vi "main OP500.vi"() -> ()   [LabVIEW 2020]
uses:
  SubVI/OP500Z8_state.ctl
  ZEN8 Semi Auto EMC/OP700/SubVI/FGV/FGV_Enum.ctl
  C:/Users/elhajj/OneDrive - FORSEE POWER/Bureau/Support banc de test/Ligne ZENPLUS/Code LabVIEW/CODE/02 SLIM ZEN WS 500/SubVi/FGV.ctl
  <userlib>/PCAN Basic/Controls/BaudrateEenum.ctl
  <userlib>/PCAN Basic/Controls/Channel.ctl
  13eb9333-f902-445b-951f-98894687dcd3.vi
  4a804ed1-565a-41e0-a699-ae70de0a1211.vi
  VG/VG_progressBar.vi
  VG/VG_Barre_Progression_ISO.vi
  DiagTool/RAMPAGE V1.0/VI/CheminDeBase.vi
  VG/VG_DCIR+OUIouNON.vi
  VG/VG_OCV70min.vi
  VG/VG_OCV70max.vi
  VG/VG_OCV30max.vi
  VG/VG_OCV30min.vi
  VG/IS30%.vi
  VG/VG_ISOmin.vi
  VG/VG_DCIRmax.vi
  VG/VG_DCIRmin.vi
  <userlib>/PCAN Basic/PCANBasic.lvlib
  <userlib>/Alex_Peak_lib/PEAK_lib_ALEX.lvlib
  <vilib>/Utility/file.llb/Read Delimited Spreadsheet (string).vi
panel:
  out "Boolean":bool
  out "DCIR+ ?":bool
  out "Barre de progression ISO":dbl(slide) scale=0.0..100.0
  out "VISA OUT":T1
  out "IS30% ?":bool
  out "Cluster":T2
  out "progression":dbl(slide) scale=0.0..100.0
  out "errout":errorcluster caption="sortie d'erreur"
  out "STOP":bool
  out "TOP":string
  out "DRAW":picture
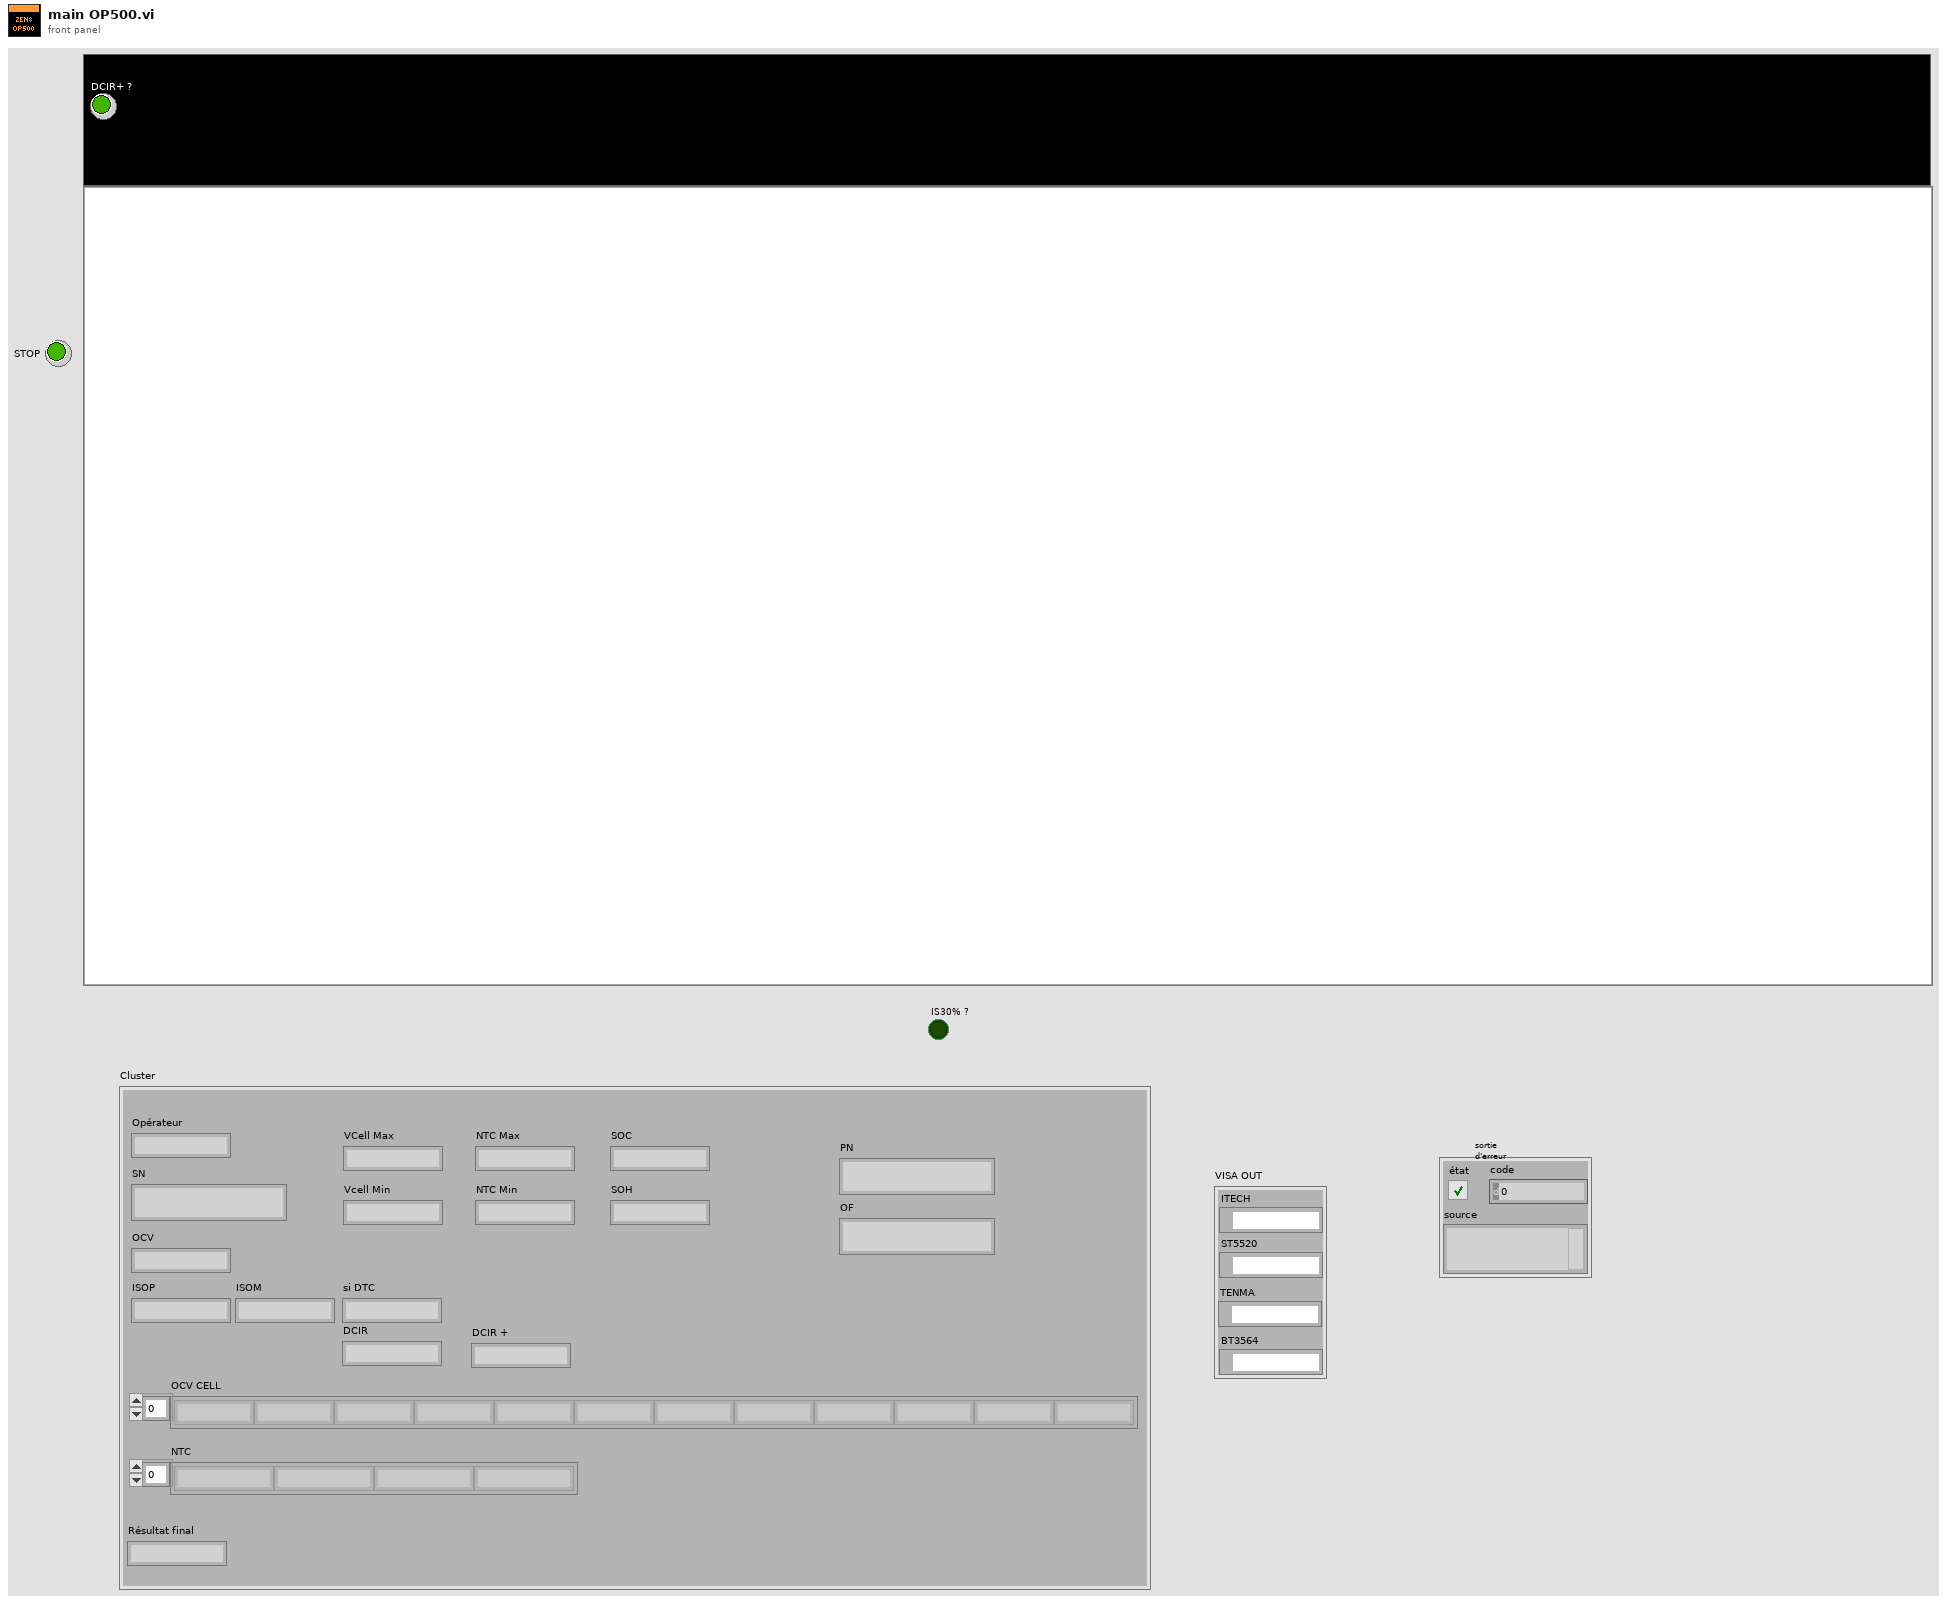
[diagram p1: front panel]
types:
  T1 = cluster{"ITECH":refnum<visa-resource-name>, "ST5520":refnum<visa-resource-name>, "TENMA":refnum<visa-resource-name>, "BT3564":refnum<visa-resource-name>}
  T2 = cluster{"Opérateur":string, "OCV":string, "ISOP":string, "ISOM":string, "Résultat final":string, "SN":string, "OCV CELL":string[], "NTC":string[], "DCIR":string, "si DTC":string, "Vcell Min":string, "VCell Max":string, "NTC Max":string, "NTC Min":string, "SOC":string, "SOH":string, "PN":string, "OF":string, "DCIR +":string}
  T3 = typedef "FGV_Enum.ctl" = enum16{"GET", "SET"}
  T4 = typedef "OP500Z8_state.ctl" = enum16{"Null", "Demarrage", "Init", "Scan", "Montage", "OCV", "Iso", "DataDyn", "Demontage", "Crash", "Next", "GoDCIR", "DCIR", "EXIT", "LogErr", "DTC"}
  T5 = typedef "FGV.ctl" = enum16{"GET", "SET", "RAZ"}
  T6 = cluster{"OCV":string, "Current":string, "VCell Max":string, "VCell Min":string, "NTC Max":string, "NTC Min":string, "SOC":string, "SOH":string, "DTC":string, "DCIR -":string, "DCIR +":string}
  T7 = cluster{"Opérateur":string, "OCV":string, "ISOP":string, "ISOM":string, "Résultat final":string, "SN":string, "OCV CELL":string[], "NTC":string[], "DCIR":string, "si DTC":string, "Vcell Min":string, "VCell Max":string, "NTC Max":string, "NTC Min":string, "SOC":string, "SOH":string, "PN":string, "OF":string, "DCIR+":string}
  T8 = typedef "imagedata.ctl" = cluster{"image type":i32, "image depth":i32, "image":u8[], "mask":u8[], "colors":u32[], "Rectangle":cluster{"left":i16, "top":i16, "right":i16, "bottom":i16}}
  T9 = typedef "PCANBasic.lvlib/Channel.ctl" = enum16{"PCAN_NONEBUS", "not used1", "not used2", "not used3", "not used4", "not used5", "not used6", "not used7", "not used8", "not used9", "not used10", "not used11", "not used12", "not used13", "not used14", "not used15", "not used16", "not used17", "not used18", "not used19", "not used20", "not used21", "not used22", "not used23", "not used24", "not used25", "not used26", "not used27", "not used28", "not used29", "not used30", "not used31", "not used32", "PCAN_ISABUS1", "PCAN_ISABUS2", "PCAN_ISABUS3", "PCAN_ISABUS4", "PCAN_ISABUS5", "PCAN_ISABUS6", "PCAN_ISABUS7", "PCAN_ISABUS8", "not used41", "not used42", "not used43", "not used44", "not used45", "not used46", "not used47", "not used48", "PCAN_DNGBUS1", "not used50", "not used51", "not used52", "not used53", "not used54", "not used55", "not used56", "not used57", "not used58", "not used59", "not used60", "not used61", "not used62", "not used63", "not used64", "PCAN_PCIBUS1", "PCAN_PCIBUS2", "PCAN_PCIBUS3", "PCAN_PCIBUS4", "PCAN_PCIBUS5", "PCAN_PCIBUS6", "PCAN_PCIBUS7", "PCAN_PCIBUS8", "not used73", "not used74", "not used75", "not used76", "not used77", "not used78", "not used79", "not used80", "PCAN_USBBUS1", "PCAN_USBBUS2", "PCAN_USBBUS3", "PCAN_USBBUS4", "PCAN_USBBUS5", "PCAN_USBBUS6", "PCAN_USBBUS7", "PCAN_USBBUS8", "Not used89", "Not used90", "Not used91", "Not used92", "Not used93", "Not used94", "Not used95", "Not used96", "PCAN_PCCBUS1", "PCAN_PCCBUS2"}
  T10 = typedef "PCANBasic.lvlib/BaudrateEenum.ctl" = enum16{"CAN_Baud_1M", "CAN_Baud_800K", "CAN_BAUD_500K", "CAN_BAUD_250K", "CAN_BAUD_125K", "CAN_BAUD_100K", "CAN_BAUD_95K", "CAN_BAUD_83K", "CAN_BAUD_50K", "CAN_BAUD_47K", "CAN_BAUD_33K", "CAN_BAUD_20K", "CAN_BAUD_10K", "CAN_BAUD_5K", "User Baudrate"}
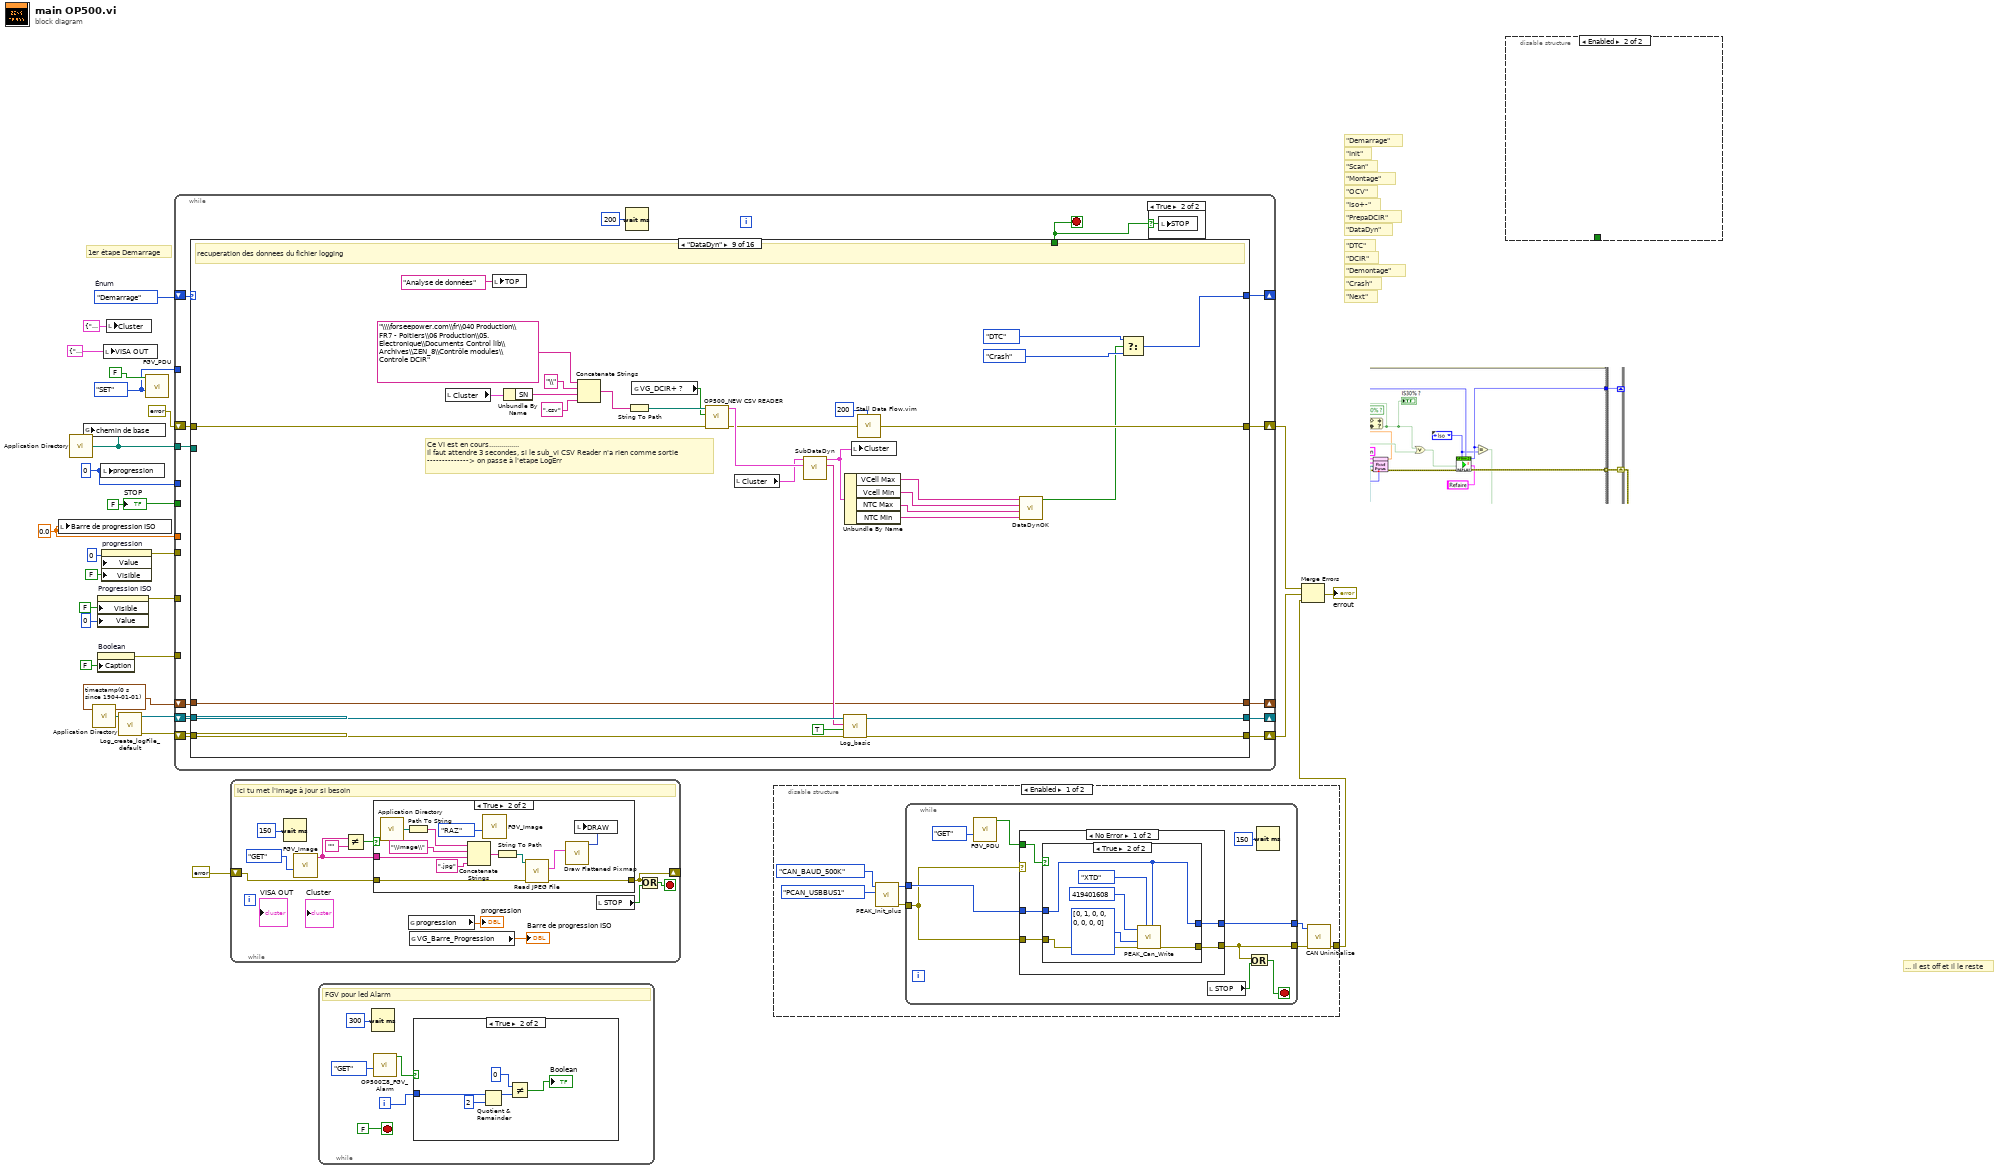
[diagram p0: block diagram]
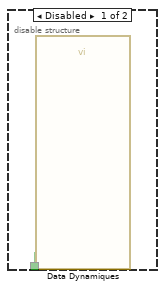
[diagram p6: hidden frame]
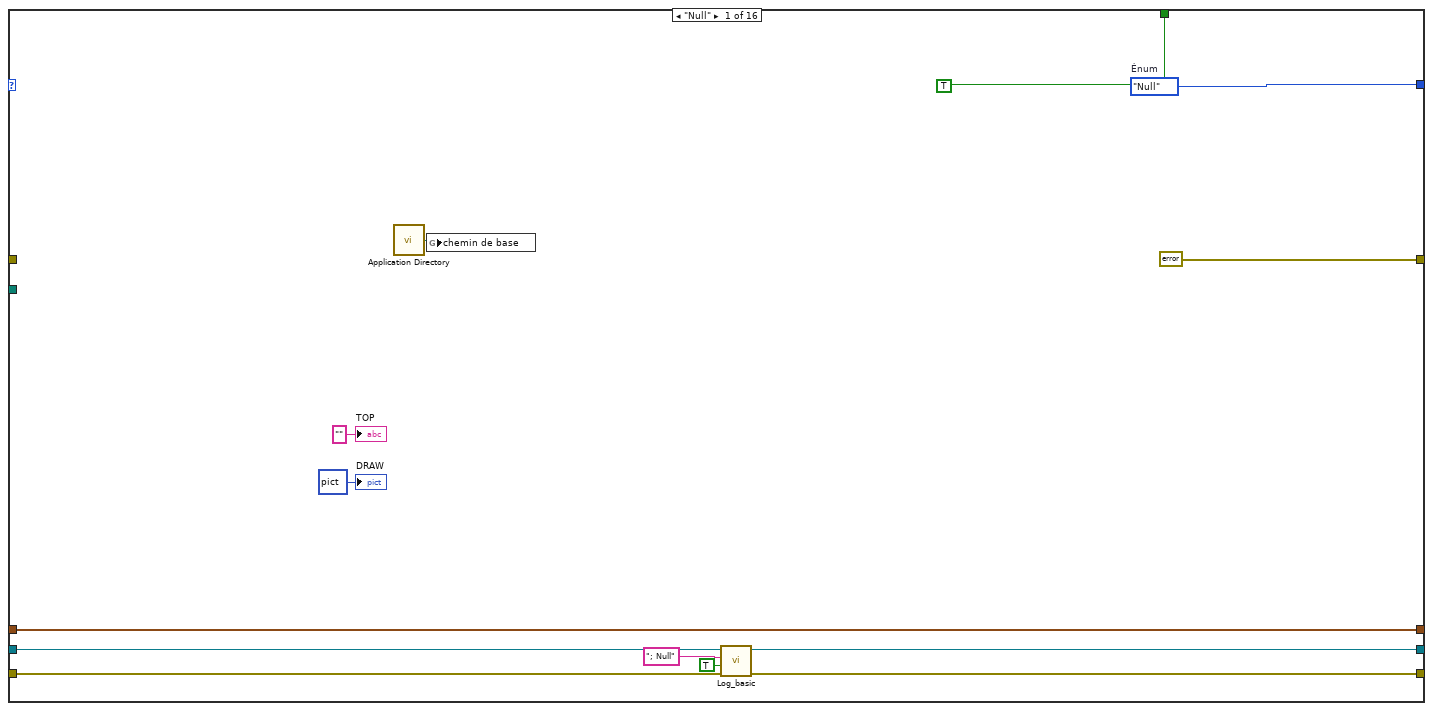
[diagram p9: hidden frame]
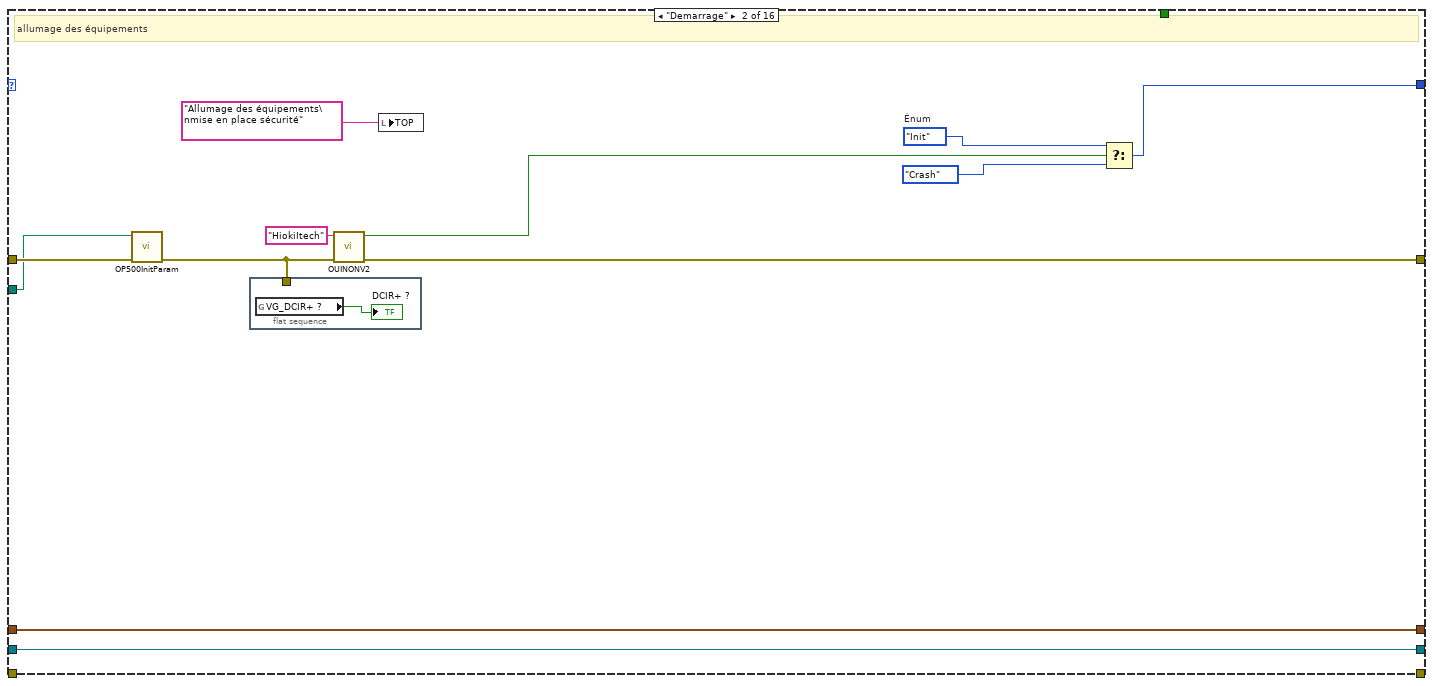
[diagram p10: hidden frame]
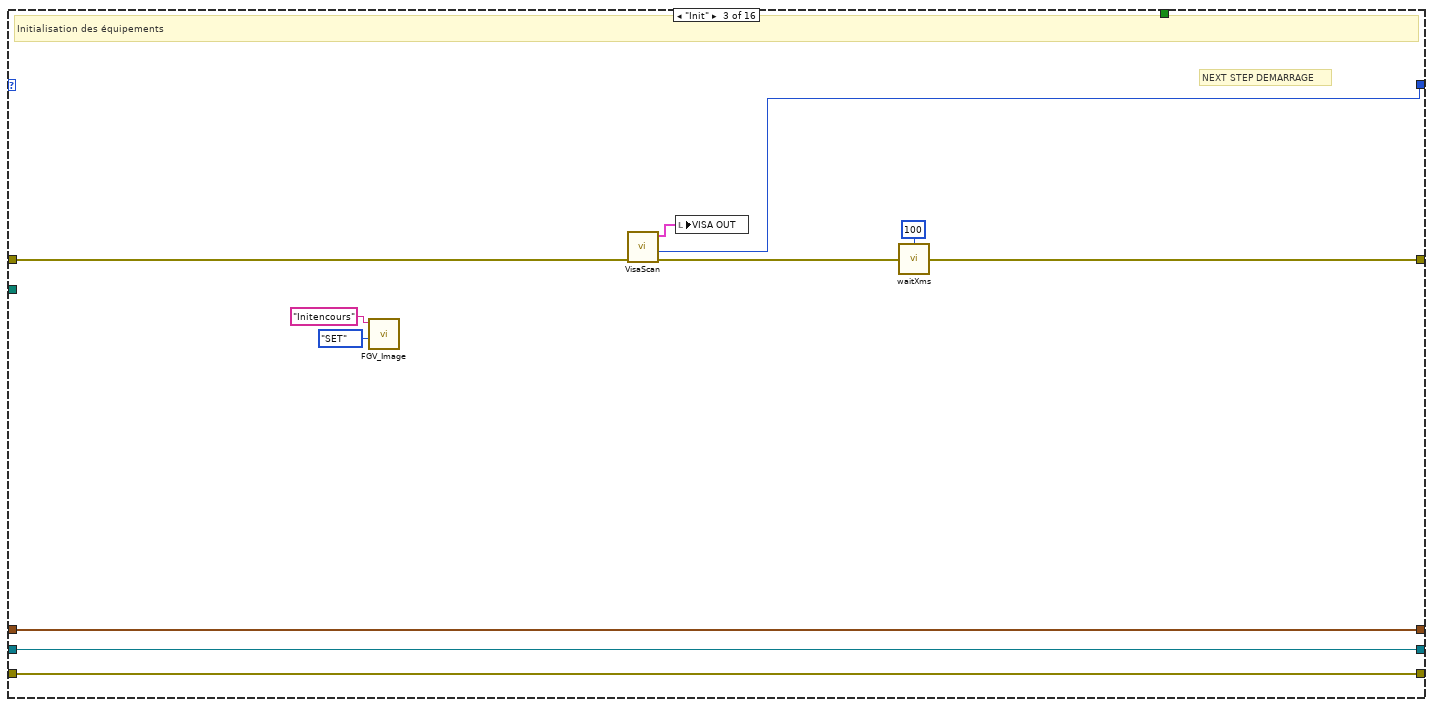
[diagram p11: hidden frame]
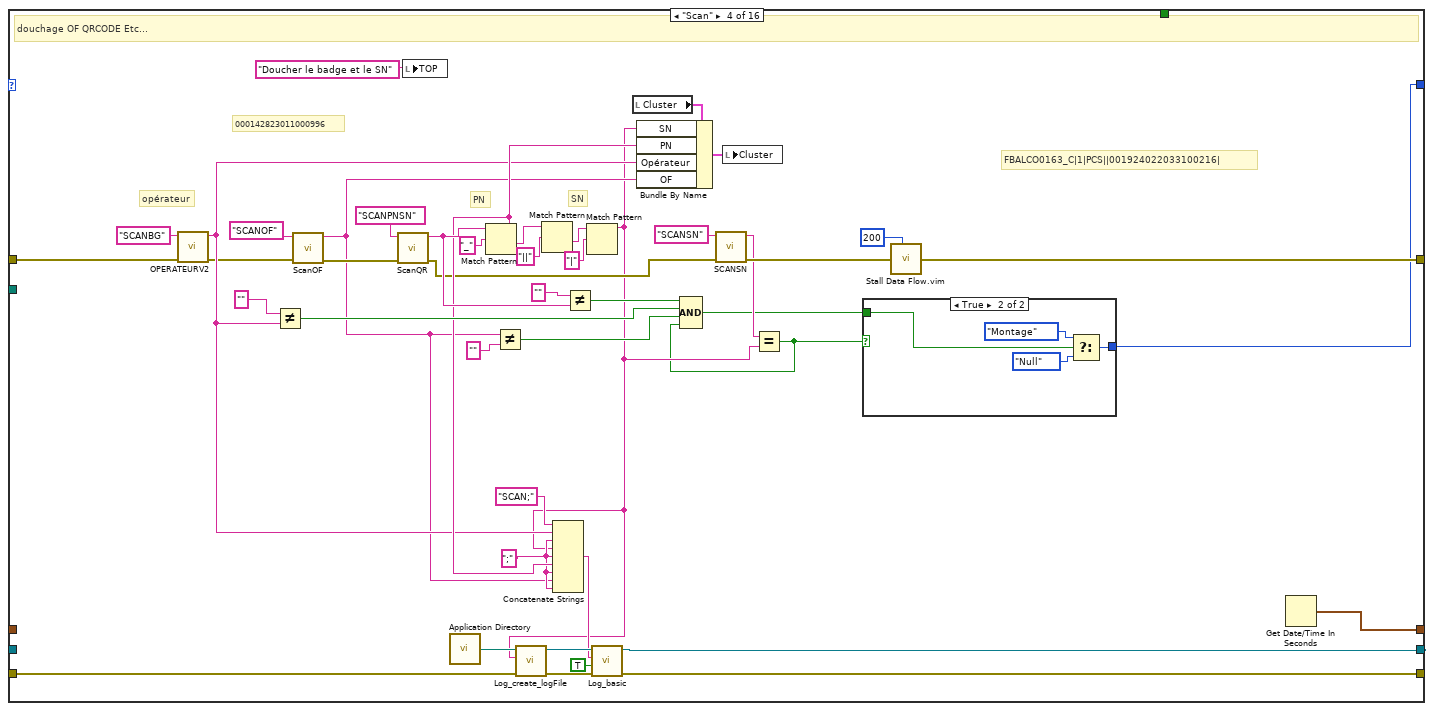
[diagram p12: hidden frame]
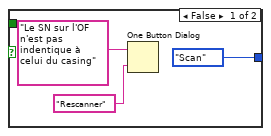
[diagram p13: hidden frame]
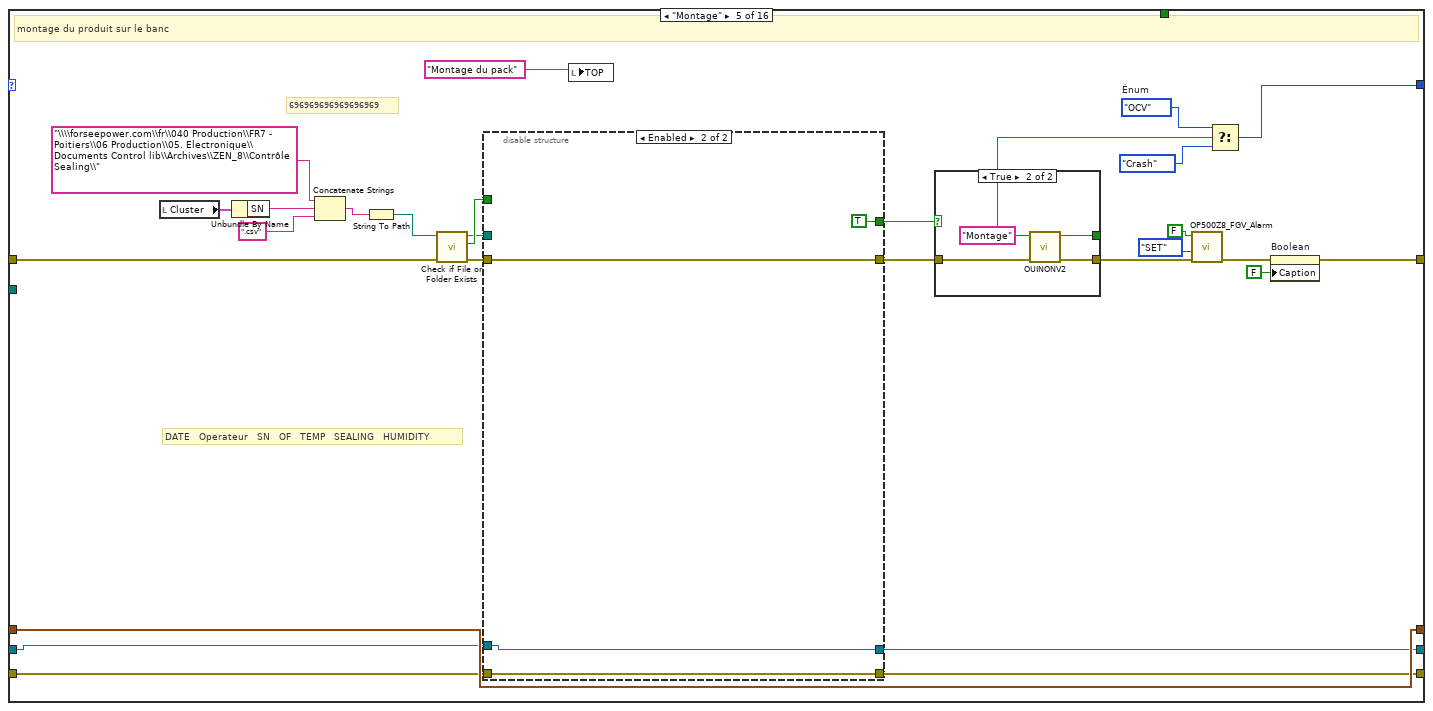
[diagram p14: hidden frame]
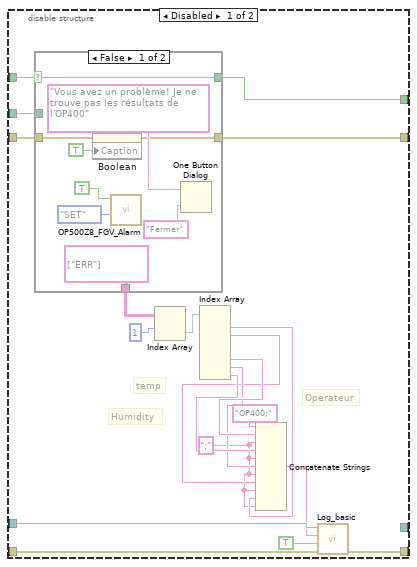
[diagram p15: hidden frame]
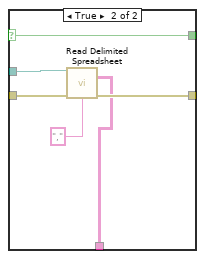
[diagram p16: hidden frame]
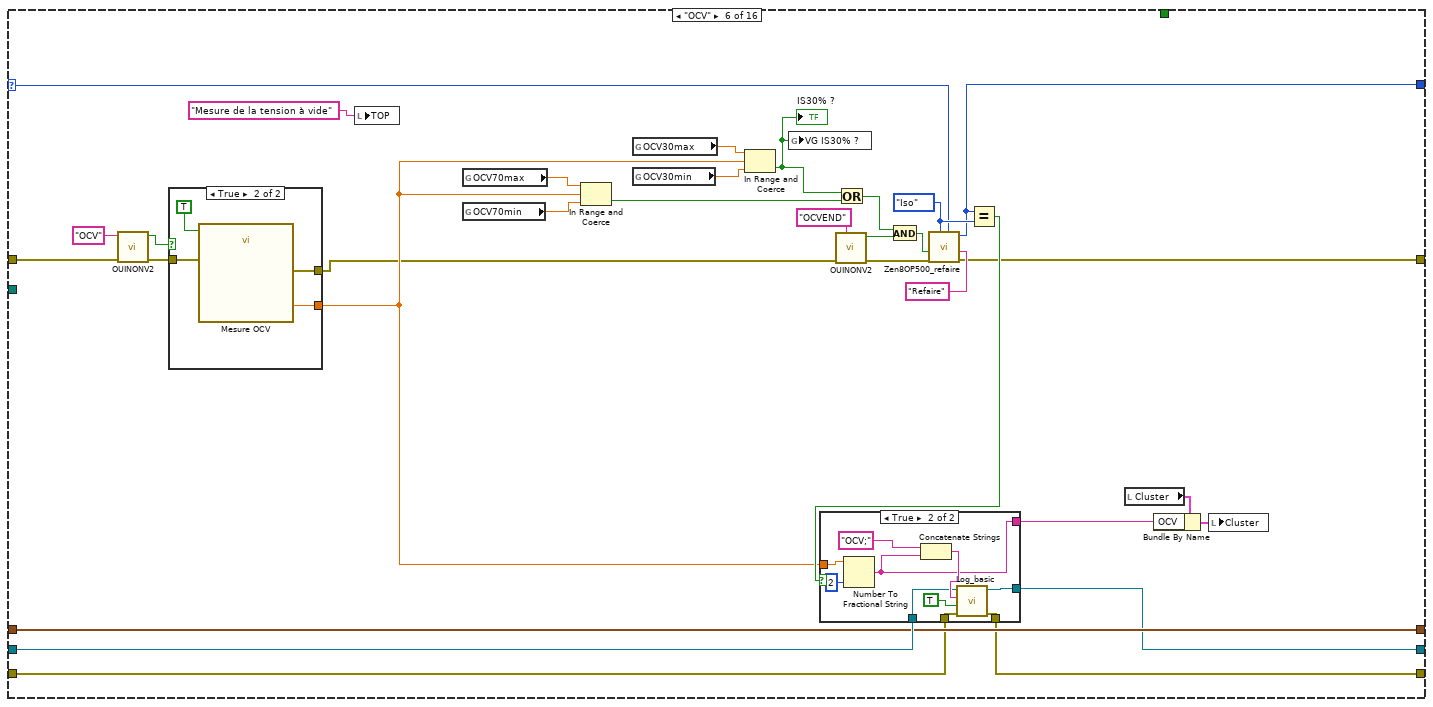
[diagram p18: hidden frame]
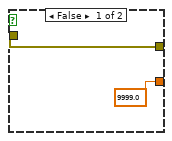
[diagram p19: hidden frame]
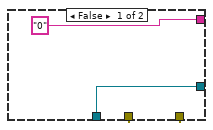
[diagram p20: hidden frame]
diagram:
  w5 = FGV_Enum."SET" ("Énum")
  w7 = 0.0 ("Barre de progression ISO")
  w17 = u8 0 ("progression")
  w12 = OP500Z8_state."Demarrage"  # Énum
  w23 = FALSE ("STOP")
  # "\"Next\""
  # "\"DCIR\""
  # "\"DTC\""
  # "1er étape Demarrage"
  # "\"Crash\""
  # "\"Demontage\""
  # "\"DataDyn\""
  # "\"Iso+-\""
  # "\"Montage\""
  # "\"Scan\""
  # "\"Init\""
  # "\"Demarrage\""
  # "\"OCV\""
  # "\"PrepaDCIR\""
  # "... il est off et il le reste"
  n1 = local write "Barre de progression ISO"(w7) -> ()
  n2 = call <vilib>:"Application Directory.vi"() -> ("Application Directory"=w22:path)
  n3 = global write "CheminDeBase.vi" "chemin de base"(w22) -> ()
  n4 = call <vilib>:"Application Directory.vi"() -> ("Application Directory"=w20:path)
  n5 = property on="Progression ISO" class="Slide (strict)"("Visible"=FALSE, "Value"=u8 0 ("Glissière")) -> (error out=w8:errorcluster)  [unwired: 2 in, 1 out]
  n6 = property on="Boolean" class="Bool (strict)"("Caption"=FALSE) -> (error out=w1:errorcluster)  [unwired: 2 in, 1 out]
  n7 = local write "progression"(w17) -> ()
  n8 = property on="progression" class="Slide (strict)"("Value"=u8 0 ("progression"), "Visible"=FALSE) -> (error out=w15:errorcluster)  [unwired: 2 in, 1 out]
  n9 = local write "VISA OUT"(T1 {"ITECH"="", "ST5520"="", "TENMA"="", "BT3564"=""} ("VISA OUT")) -> ()
  n10 = local write "Cluster"(T2 {"Opérateur"="", "OCV"="", "ISOP"="", "ISOM"="", "Résultat final"="", "SN"="", "OCV CELL"=[], "NTC"=[], "DCIR"="", "si DTC"="", "Vcell Min"="", "VCell Max"="", "NTC Max"="", "NTC Min"="", "SOC"="", "SOH"="", "PN"="", "OF"="", "DCIR +"=""} ("Cluster")) -> ()
  n11 = call <userlib>:"Log_create_logFile_default.vi"("appdir"=w20) -> ("errout"=w21:errorcluster, "Fichier à flux d'octets en sortie"=w24:refnum<file>)  [unwired: 9 in]
  n12 = call "FGV_PDU.vi"("Énum"=w5, "IN"=FALSE) -> ()  [unwired: 8 in, 2 out]
  n13 = while {
    shift-right: [w39] -> w26
    shift-left: errorcluster {"status"=FALSE, "code"=0, "source"=""} ("error out") -> [w30]
    shift-right: [w35] -> w25
    shift-left: w21 -> [w38]
    shift-right: [w36] -> _
    shift-left: w24 -> [w37]
    tunnel: w22 -> [w33]
    tunnel: w23 -> [_]
    shift-right: [w31] -> _
    shift-left: timestamp(0 s since 1904-01-01) ("seconds since 1Jan1904") -> [w32]
    tunnel: w17 -> [_]
    tunnel: w15 -> [_]
    shift-right: [w28] -> _
    shift-left: w12 -> [w29]
    tunnel: w8 -> [_]
    tunnel: w7 -> [_]
    tunnel: w5 -> [_]
    tunnel: w1 -> [_]
    stop <- w34 stop-if-true
    n14 = case "Structure Condition" shown="\"DataDyn\"" w29 {
      selector: w29 -> [_ _ _ _ _ w223 _ _ _ _ _ _ _ _ _ _]
      tunnel: w30 -> [_ w59 w73 w123 w146 w221 w272 w364 w479 w502 w528 w550 w566 w588 w640 w646]
      tunnel: [errorcluster {"status"=FALSE, "code"=0, "source"=""} ("errin") w56 w69 w89 w137 w217 w290 w359 w473 w501 w527 w544 w566 w577 w639 w647] -> w39
      tunnel: w38 -> [w50 _ w78 w119 w136 w230 w300 w365 w488 w510 w535 w552 w569 w603 _ _]
      tunnel: w37 -> [w51 w66 w77 _ w134 w232 w299 w366 w486 w509 w540 w553 w570 w604 _ _]
      tunnel: [w48 w66 w77 w121 w131 w228 w298 w366 w485 w508 w541 w553 _ _ _ _] -> w36
      tunnel: [w49 _ w78 w122 w135 w229 w301 w365 w487 w510 w542 w552 w557 w592 _ _] -> w35
      tunnel: [TRUE _ _ _ _ _ _ _ _ _ _ FALSE w571 _ _ _] -> w34
      tunnel: w33 -> [_ w58 _ _ _ _ w270 _ _ _ _ _ _ _ _ _]
      tunnel: w32 -> [w44 w65 w76 _ w158 w231 w295 w368 w478 _ _ w549 _ _ _ _]
      tunnel: [w44 w65 w76 w110 w158 w231 w295 w368 w478 _ _ w549 _ _ _ _] -> w31
      tunnel: [w42 w60 w72 w80 w153 w222 w279 w363 w465 w494 w530 w545 OP500Z8_state."Crash" w593 w636 w648] -> w28
      frame "Null" {
        w42 = OP500Z8_state."Null"  # Énum
        n15 = call <vilib>:"Application Directory.vi"() -> ("Application Directory"=w54:path)
        n16 = global write "CheminDeBase.vi" "chemin de base"(w54) -> ()
        n17 = call <userlib>:"Log_basic.vi"("errin"=w50, "date?"=TRUE, "chaîne"="; Null", "in"=w51) -> ("sortie d'erreur"=w49:errorcluster, "refnum en sortie"=w48:refnum<file>)  [unwired: 6 in]
        "DRAW" <- picture data[5B] ("DRAW")
        "TOP" <- "" ("TOP")
      }
      frame "Demarrage" {
        w62 = OP500Z8_state."Init"  # Énum
        # "allumage des équipements"
        n18 = call "OP500InitParam.vi"("errin"=w59, "pathin"=w58) -> ("errout"=w55:errorcluster)  [unwired: 9 in]
        n19 = flat-sequence {
          tunnel: w55 -> [_]
          frame #0 {
            n20 = global read "VG_DCIR+OUIouNON.vi" "VG_DCIR+ ?"() -> (→"DCIR+ ?":bool)
          }
        }
        n21 = call "OUINONV2.vi"("errin"=w55, "image"="HiokiItech") -> ("error out"=w56:errorcluster, "Booléen"=w57:bool)  [unwired: 8 in]
        n22 = local write "TOP"("Allumage des équipements\nmise en place sécurité" ("TOP")) -> ()
        n23 = Select ("Sélectionner")(t=w62, s=w57, f=OP500Z8_state."Crash" ("cas faux")) -> (s? t:f=w60:T4)
      }
      frame "Init" {
        # "NEXT STEP DEMARRAGE"
        # "Initialisation des équipements"
        n24 = call "FGV_Image.vi"("Énum"=FGV."SET", "IN"="Initencours") -> ()  [unwired: 9 in, 1 out]
        n25 = call "VisaScan.vi"("errin"=w73) -> ("errout"=w70:errorcluster, "NextStep"=w72:T4, "VISA OUT"=w68:T1)  [unwired: 8 in]
        n26 = local write "VISA OUT"(w68) -> ()
        n27 = call <userlib>:"waitXms.vi"("attente (ms)"=u32 100, "errin"=w70) -> ("errout"=w69:errorcluster)  [unwired: 13 in]
      }
      frame "Scan" {
        w93 = ";" ("chaîne")
        # "SN"
        # "PN"
        # "FBALCO0163_C|1|PCS||001924022033100216|"
        # "000142823011000996"
        # "opérateur"
        # "douchage OF QRCODE Etc..."
        n28 = call "OPERATEURV2.vi"("errin"=w123, "IN"="SCANBG") -> ("error out"=w92:errorcluster, "Dataout"=w97:string)  [unwired: 8 in]
        n29 = Not Equal?(x="", y=w97) -> (x != y?=w111:bool)
        n30 = call <userlib>:"ScanOF.vi"("errin"=w92, "image"="SCANOF") -> ("error out"=w91:errorcluster, "OF"=w87:string)  [unwired: 8 in]
        n31 = call <userlib>:"ScanQR.vi"("errin"=w91, "image"="SCANPNSN") -> ("error out"=w86:errorcluster, "OF"=w104:string)  [unwired: 7 in, 1 out]
        n32 = local write "TOP"("Doucher le badge et le SN" ("TOP")) -> ()
        n33 = call <vilib>:"Application Directory.vi"() -> ("Application Directory"=w120:path)
        n34 = Match Pattern(string=w104, regular expression="_" ("expression régulière")) -> (before substring=w98:string, after substring=w102:string)  [unwired: 1 in, 2 out]
        n35 = Not Equal?(x=w87, y="") -> (x != y?=w94:bool)
        n36 = Match Pattern(string=w102, regular expression="||" ("expression régulière")) -> (after substring=w100:string)  [unwired: 1 in, 3 out]
        n37 = Not Equal?(x="", y=w104) -> (x != y?=w112:bool)
        n38 = Match Pattern(string=w100, regular expression="|" ("expression régulière")) -> (before substring=w82:string)  [unwired: 1 in, 3 out]
        n39 = call <userlib>:"Log_create_logFile.vi"("errin"=w119, "toute l'expression"=w82, "Application Directory"=w120) -> ("sortie d'erreur"=w117:errorcluster, "Fichier à flux d'octets en sortie"=w118:refnum<file>)  [unwired: 7 in]
        n40 = Concatenate Strings("SCAN;" ("chaîne"), w97, w93, w82, w93, w98, w93, w87, w93) -> (w115:string)
        n41 = call <userlib>:"Log_basic.vi"("errin"=w117, "date?"=TRUE, "chaîne"=w115, "in"=w118) -> ("sortie d'erreur"=w122:errorcluster, "refnum en sortie"=w121:refnum<file>)  [unwired: 6 in]
        n42 = local read "Cluster"() -> (w106:T2)
        n43 = Bundle By Name(cluster=w106, "SN"=w82, "PN"=w98, "Opérateur"=w97, "OF"=w87) -> (w105:T2)
        n44 = call <userlib>:"SCANSN.vi"("errin"=w86, "image"="SCANSN") -> ("error out"=w85:errorcluster, "SN"=w83:string)  [unwired: 8 in]
        n45 = local write "Cluster"(w105) -> ()
        n46 = Equal?(x=w83, y=w82) -> (x = y?=w81:bool)
        n47 = Compound Arithmetic op=AND ("Opérateur arithmétique")(w112, w111, w94, w81) -> (w79:bool)
        n48 = case shown="True" w81 {
          tunnel: [OP500Z8_state."Scan" ("cas faux") w128] -> w80
          tunnel: w79 -> [_ w127]
          frame False {
            n49 = One Button Dialog(message="Le SN sur l'OF n'est pas indentique à celui du casing", button name ("OK")="Rescanner" ("nom du bouton (\"OK\")")) -> ()  [unwired: 1 out]
          }
          frame True {
            n50 = Select ("Sélectionner")(t=OP500Z8_state."Montage" ("Énum"), s=w127, f=OP500Z8_state."Null" ("cas faux")) -> (s? t:f=w128:T4)
          }
        }
        n51 = call "Stall Data Flow.vim"("value in"=w85, "milliseconds to wait"=u32 200) -> ("value out"=w89:errorcluster)  [unwired: 1 out]
        n52 = Get Date/Time In Seconds() -> (seconds since 1Jan1904=w110:timestamp)
      }
      frame "Montage" {
        w156 = OP500Z8_state."OCV"  # Énum
        # "DATE   Operateur   SN   OF   TEMP   SEALING   HUMIDITY"
        # "696969696969696969"
        # "montage du produit sur le banc"
        n53 = local read "Cluster"() -> (w152:T2)
        n54 = Unbundle By Name(w152) -> ("SN"=w151:string)
        n55 = Concatenate Strings("\\\\forseepower.com\\fr\\040 Production\\FR7 - Poitiers\\06 Production\\05. Electronique\\Documents Control lib\\Archives\\ZEN_8\\Contrôle Sealing\\" ("string"), w151, ".csv" ("string")) -> (w148:string)
        n56 = String To Path(string=w148) -> (path=w147:path)
        n57 = call <vilib>:"Check if File or Folder Exists.vi"("error in (no error)"=w146, "path"=w147) -> ("error out"=w145:errorcluster, "file or folder exists?"=w144:bool, "dup path"=w143:path)  [unwired: 7 in]
        n58 = disable-structure shown="Enabled" {
          disable-tunnel: w145 -> [w178 w197]
          disable-tunnel: w144 -> [w177 _]
          disable-tunnel: w143 -> [w176 _]
          disable-tunnel: w136 -> [w175 w195]
          disable-tunnel: [w174 w195] -> w135
          disable-tunnel: w134 -> [w173 w194]
          disable-tunnel: [w172 w197] -> w133
          disable-tunnel: [w171 TRUE] -> w132
          disable-tunnel: [_ w194] -> w131
          frame Disabled {
            w159 = ";" ("string")
            # "Operateur"
            # "Humidity"
            # "temp"
            n59 = case shown="False" w177 {
              selector: w177 -> [w187 w190]
              tunnel: [w182 w192] -> w172
              tunnel: w178 -> [w183 w191]
              tunnel: [w187 w190] -> w171
              tunnel: w176 -> [_ w189]
              tunnel: [string[][] [["ERR"]] ("all rows") w188] -> w166
              frame False {
                n60 = property on="Boolean" class="Bool (strict)"(error in=w183, "Caption"=TRUE) -> (error out=w182:errorcluster)  [unwired: 1 in, 1 out]
                n61 = call "OP500Z8_FGV_Alarm.vi"("Énum"=FGV_Enum."SET", "IN"=TRUE) -> ()  [unwired: 8 in, 2 out]
                n62 = One Button Dialog(message="Vous avez un problème! Je ne trouve pas les résultats de l'OP400", button name ("OK")="Fermer") -> ()  [unwired: 1 out]
              }
              frame True {
                n63 = call-poly <vilib>:"Read Delimited Spreadsheet.vi"("file path (dialog if empty)"=w189, "error in (no error)"=w191, "delimiter (\\t)"="," ("delimiter (\\t)")) -> ("all rows"=w188:string[][], "error out"=w192:errorcluster)  [unwired: 7 in, 4 out]
              }
            }
            n64 = Index Array(array=w166, index (row)=1) -> (element=w165:string[])  [unwired: 1 in]
            n65 = Index Array(array=w165) -> (element #1=w160:string, element #2=w161:string, element #5=w163:string, element #6=w162:string, element #7=w164:string)  [unwired: 7 in, 2 out]
            n66 = Concatenate Strings("OP400;" ("string"), w163, w159, w164, w159, w162, w159, w161, w159, w160, w159) -> (w169:string)
            n67 = call <userlib>:"Log_basic.vi"("errin"=w175, "date?"=TRUE, "chaîne"=w169, "in"=w173) -> ("sortie d'erreur"=w174:errorcluster)  [unwired: 6 in, 1 out]
          }
          frame Enabled {
          }
        }
        n68 = local write "TOP"("Montage du pack" ("TOP")) -> ()
        n69 = case shown="True" w132 {
          selector: w132 -> [w198 _]
          tunnel: [w199 w202] -> w142
          tunnel: [w198 w201] -> w157
          tunnel: w133 -> [w199 w200]
          frame False {
          }
          frame True {
            n70 = call "OUINONV2.vi"("errin"=w200, "image"="Montage" ("IN")) -> ("error out"=w202:errorcluster, "Booléen"=w201:bool)  [unwired: 8 in]
          }
        }
        n71 = call "OP500Z8_FGV_Alarm.vi"("errin"=w142, "Énum"=FGV_Enum."SET", "IN"=FALSE) -> ("errout"=w138:errorcluster)  [unwired: 7 in, 1 out]
        n72 = Select ("Sélectionner")(t=w156, s=w157, f=OP500Z8_state."Crash" ("cas faux")) -> (s? t:f=w153:T4)
        n73 = property on="Boolean" class="Bool (strict)"(error in=w138, "Caption"=FALSE) -> (error out=w137:errorcluster)  [unwired: 1 in, 1 out]
      }
      frame "OCV" {
        w234 = OP500Z8_state."Iso" ("Cas OK")
        n74 = call "OUINONV2.vi"("errin"=w221, "image"="OCV" ("IN")) -> ("error out"=w220:errorcluster, "Booléen"=w218:bool)  [unwired: 8 in]
        n75 = case shown="True" w218 {
          tunnel: [w237 w241] -> w213
          tunnel: [9999.0 ("Tension Bat+ Bat-") w239] -> w216
          tunnel: w220 -> [w237 w238]
          frame False {
          }
          frame True {
            n76 = call "Mesure OCV"("Enable"=TRUE, "error in (no error)"=w238) -> ("Tension Bat+ Bat-"=w239:dbl, "error out"=w241:errorcluster)  [unwired: 15 in, 1 out]
          }
        }
        n77 = local write "TOP"("Mesure de la tension à vide" ("TOP")) -> ()
        n78 = global read "VG_OCV70max.vi" "OCV70max"() -> (w207:dbl)
        n79 = global read "VG_OCV70min.vi" "OCV70min"() -> (w206:dbl)
        n80 = In Range and Coerce(upper limit=w207, x=w216, lower limit=w206) -> (In Range?=w215:bool)  [unwired: 1 out]
        n81 = global read "VG_OCV30max.vi" "OCV30max"() -> (w205:dbl)
        n82 = global read "VG_OCV30min.vi" "OCV30min"() -> (w204:dbl)
        n83 = In Range and Coerce(upper limit=w205, x=w216, lower limit=w204) -> (In Range?=w214:bool)  [unwired: 1 out]
        "IS30% ?" <- w214
        n84 = global write "IS30%.vi" "VG IS30% ?"(w214) -> ()
        n85 = call "OUINONV2.vi"("errin"=w213, "image"="OCVEND" ("IN")) -> ("error out"=w211:errorcluster, "Booléen"=w210:bool)  [unwired: 8 in]
        n86 = Or(x=w214, y=w215) -> (x .or. y?=w208:bool)
        n87 = And(x=w208, y=w210) -> (x .and. y?=w209:bool)
        n88 = call "Zen8OP500_refaire.vi"("image"="Refaire", "refaire"=w223, "casOK"=w234, "errin"=w211, "test ok ?"=w209) -> ("errout"=w217:errorcluster, "Next"=w222:T4)  [unwired: 5 in]
        n89 = Equal?(x=w222, y=w234) -> (x = y?=w233:bool)
        n90 = case shown="True" w233 {
          tunnel: w230 -> [w244 w251]
          tunnel: [w244 w250] -> w229
          tunnel: w232 -> [w243 w249]
          tunnel: [w243 w248] -> w228
          tunnel: w216 -> [_ w247]
          tunnel: ["0" w246] -> w224
          frame False {
          }
          frame True {
            n91 = Number To Fractional String(number=w247, precision (6)=i16 2 ("précision (6)")) -> (F-format string=w246:string)  [unwired: 2 in]
            n92 = Concatenate Strings("OCV;" ("chaîne"), w246) -> (w253:string)
            n93 = call <userlib>:"Log_basic.vi"("errin"=w251, "date?"=TRUE, "chaîne"=w253, "in"=w249) -> ("sortie d'erreur"=w250:errorcluster, "refnum en sortie"=w248:refnum<file>)  [unwired: 6 in]
          }
        }
        n94 = local read "Cluster"() -> (w226:T2)
        n95 = Bundle By Name(cluster=w226, "OCV"=w224) -> (w225:T2)
        n96 = local write "Cluster"(w225) -> ()
      }
      frame "Iso" {
        # "test d'isolement Bat+ et Bat-"
        n97 = call "OUINONV2.vi"("errin"=w272, "image"="ISOSTART") -> ("error out"=w277:errorcluster, "Booléen"=w275:bool)  [unwired: 8 in]
        n98 = case shown="True" w275 {
          selector: w275 -> [w308 _]
          tunnel: [w309 w313] -> w283
          tunnel: [w308 w311] -> w282
          tunnel: w277 -> [w309 w310]
          frame False {
          }
          frame True {
            n99 = call "OUINONV2.vi"("errin"=w310, "image"="MultiEPI") -> ("error out"=w313:errorcluster, "Booléen"=w311:bool)  [unwired: 8 in]
          }
        }
        n100 = local read "VISA OUT"() -> (w269:T1)
        n101 = case shown="True" w282 {
          selector: w282 -> [w314 _]
          tunnel: [w314 w318] -> w285
          tunnel: [w315 w317] -> w260
          tunnel: w283 -> [w315 w316]
          frame False {
          }
          frame True {
            n102 = call "OUINONV2.vi"("errin"=w316, "image"="ISOP" ("IN")) -> ("error out"=w317:errorcluster, "Booléen"=w318:bool)  [unwired: 8 in]
          }
        }
        n103 = Unbundle By Name(w269) -> ("ST5520"=w268:refnum<visa-resource-name>)
        n104 = global read "VG_ISOmin.vi" "Iso"() -> (w278:dbl)
        n105 = property on="PB ISO" class="Slide (strict)"(error in=w260, "Visible"=TRUE) -> (error out=w259:errorcluster)  [unwired: 1 in, 1 out]
        n106 = local write "TOP"("Test d'isolement Bat+" ("TOP")) -> ()
        n107 = case shown="True" w285 {
          selector: w285 -> [w337 _]
          tunnel: w259 -> [w338 w346]
          tunnel: [w338 w345] -> w266
          tunnel: [w336 w348] -> w297
          tunnel: [w337 w349] -> w289
          tunnel: w278 -> [_ w339]
          tunnel: [w336 w348] -> w292
          tunnel: w270 -> [_ w347]
          tunnel: w268 -> [_ w343]
          frame False {
            w336 = "ERR"
          }
          frame True {
            w350 = i16 2 ("largeur (-)")
            n108 = call "OP500Z8_ST5520.vi"("errin"=w346, "chemin de base"=w347, "Refnum VISA en entrée"=w343) -> ("error out"=w345:errorcluster, "R iso(MOhm)"=w341:dbl)  [unwired: 7 in]
            n109 = call "FGV_Image.vi"("Énum"=FGV."SET", "IN"="IsoEnCours") -> ()  [unwired: 9 in, 1 out]
            n110 = Number To Fractional String(number=w341, width (-)=w350, precision (6)=w350) -> (F-format string=w348:string)  [unwired: 1 in]
            n111 = In Range and Coerce(upper limit=9991.0 ("limite supérieure"), x=w341, lower limit=w339) -> (In Range?=w349:bool)  [unwired: 1 out]
          }
        }
        n112 = property on="PB ISO" class="Slide (strict)"(error in=w266, "Visible"=FALSE, "Value"=u8 0 ("Barre de progression ISO")) -> (error out=w264:errorcluster)  [unwired: 1 in, 1 out]
        n113 = flat-sequence {
          tunnel: w264 -> [_]
          frame #0 {
            n114 = local write "TOP"("Test d'isolement Bat-" ("TOP")) -> ()
          }
        }
        n115 = call "OUINONV2.vi"("errin"=w264, "image"="ISOM" ("IN")) -> ("error out"=w263:errorcluster, "Booléen"=w303:bool)  [unwired: 8 in]
        n116 = local read "Cluster"() -> (w294:T2)
        n117 = property on="PB ISO" class="Slide (strict)"(error in=w263, "Visible"=TRUE) -> (error out=w262:errorcluster)  [unwired: 1 in, 1 out]
        n118 = case shown="True" w303 {
          selector: w303 -> [w323 _]
          tunnel: [w321 w332] -> w257
          tunnel: [w322 w334] -> w296
          tunnel: [w323 w327] -> w288
          tunnel: w278 -> [_ w326]
          tunnel: [w322 w334] -> w291
          tunnel: w262 -> [w321 w333]
          tunnel: w270 -> [_ w331]
          tunnel: w268 -> [_ w329]
          frame False {
            w322 = "ERR"
          }
          frame True {
            w335 = i16 2 ("largeur (-)")
            n119 = call "OP500Z8_ST5520.vi"("errin"=w333, "chemin de base"=w331, "Refnum VISA en entrée"=w329) -> ("error out"=w332:errorcluster, "R iso(MOhm)"=w325:dbl)  [unwired: 7 in]
            n120 = call "FGV_Image.vi"("Énum"=FGV."SET", "IN"="IsoEnCours") -> ()  [unwired: 9 in, 1 out]
            n121 = Number To Fractional String(number=w325, width (-)=w335, precision (6)=w335) -> (F-format string=w334:string)  [unwired: 1 in]
            n122 = In Range and Coerce(upper limit=9991.0 ("limite supérieure"), x=w325, lower limit=w326) -> (In Range?=w327:bool)  [unwired: 1 out]
          }
        }
        n123 = Bundle By Name(cluster=w294, "ISOP"=w292, "ISOM"=w291) -> (w293:T2)
        n124 = local write "Cluster"(w293) -> ()
        n125 = Concatenate Strings("Iso+;" ("chaîne"), w297, ";Iso-;" ("chaîne"), w296) -> (w307:string)
        n126 = call <userlib>:"Log_basic.vi"("errin"=w300, "date?"=TRUE, "chaîne"=w307, "in"=w299) -> ("sortie d'erreur"=w301:errorcluster, "refnum en sortie"=w298:refnum<file>)  [unwired: 6 in]
        n127 = property on="PB ISO" class="Slide (strict)"(error in=w257, "Visible"=FALSE) -> (error out=w256:errorcluster)  [unwired: 1 in, 1 out]
        n128 = call "OUINONV2.vi"("errin"=w256, "image"="EPIOFF") -> ("error out"=w274:errorcluster)  [unwired: 8 in, 1 out]
        n129 = call "OUINONV2.vi"("errin"=w274, "image"="ISOEND") -> ("error out"=w290:errorcluster, "Booléen"=w287:bool)  [unwired: 8 in]
        n130 = Compound Arithmetic op=AND ("Opérateur arithmétique")(w289, w288, w287) -> (w286:bool)
        n131 = Select ("Sélectionner")(t=OP500Z8_state."GoDCIR" ("cas vrai"), s=w286, f=OP500Z8_state."Crash" ("Énum")) -> (s? t:f=w279:T4)
      }
      frame "GoDCIR" {
        # "Lancer la DCIR : fermature des contacteurs + control ITECH + Logging"
        n132 = call "OUINONV2.vi"("errin"=w364, "image"="DCIRCABLAGE") -> ("error out"=w362:errorcluster)  [unwired: 8 in, 1 out]
        n133 = local write "TOP"("Test DCIR" ("TOP")) -> ()
        n134 = local read "VISA OUT"() -> (w358:T1)
        n135 = Unbundle By Name(w358) -> ("ITECH"=w353:refnum<visa-resource-name>, "TENMA"=w352:refnum<visa-resource-name>)
        n136 = local read "Cluster"() -> (w357:T2)
        n137 = Unbundle By Name(w357) -> ("SN"=w356:string)
        n138 = disable-structure shown="Enabled" {
          disable-tunnel: w362 -> [w383 w438]
          disable-tunnel: [w380 w445] -> w361
          disable-tunnel: [w379 w446] -> w351
          disable-tunnel: w353 -> [_ w444]
          disable-tunnel: w356 -> [_ w443]
          disable-tunnel: w353 -> [_ w442]
          disable-tunnel: w352 -> [_ w437]
          frame Disabled {
            n139 = case shown="True" {
              selector: _ -> [w401 _]
              tunnel: [w401 w404] -> w374
              tunnel: w383 -> [w400 w403]
              tunnel: [w400 w402] -> w376
              frame False {
              }
              frame True {
                n140 = call "OUINONV2.vi"("errin"=w403, "image"="BMS") -> ("error out"=w402:errorcluster, "Booléen"=w404:bool)  [unwired: 8 in]
              }
            }
            n141 = case shown="True" w374 {
              selector: w374 -> [w389 _]
              tunnel: [w389 w392] -> w373
              tunnel: w376 -> [w388 w391]
              tunnel: [w388 w390] -> w375
              frame False {
              }
              frame True {
                n142 = call "OUINONV2.vi"("errin"=w391, "image"="PCANVIEW") -> ("error out"=w390:errorcluster, "Booléen"=w392:bool)  [unwired: 8 in]
              }
            }
            n143 = case shown="True" w373 {
              selector: w373 -> [w407 _]
              tunnel: [w407 w410] -> w378
              tunnel: w375 -> [w406 w409]
              tunnel: [w406 w408] -> w377
              frame False {
              }
              frame True {
                n144 = call "OUINONV2.vi"("errin"=w409, "image"="DCIRON") -> ("error out"=w408:errorcluster, "Booléen"=w410:bool)  [unwired: 8 in]
              }
            }
            n145 = case shown="True" w378 {
              selector: w378 -> [w395 _]
              tunnel: [w394 w398] -> w387
              tunnel: [w395 w397] -> w386
              tunnel: w377 -> [w394 w396]
              frame False {
              }
              frame True {
                n146 = call "OUINONV2.vi"("errin"=w396, "image"="Logging") -> ("error out"=w398:errorcluster, "Booléen"=w397:bool)  [unwired: 8 in]
              }
            }
            n147 = case shown="True" w386 {
              selector: w386 -> [w424 _]
              tunnel: w387 -> [w425 w429]
              tunnel: [w425 w427] -> w382
              tunnel: [w424 w426] -> w385
              frame False {
              }
              frame True {
                n148 = call "OUINONV2.vi"("errin"=w429, "image"="Minuteur") -> ("error out"=w427:errorcluster, "Booléen"=w426:bool)  [unwired: 8 in]
              }
            }
            n149 = case shown="True" w385 {
              selector: w385 -> [w419 _]
              tunnel: [w419 w422] -> w384
              tunnel: w382 -> [w418 w421]
              tunnel: [w418 w420] -> w381
              frame False {
              }
              frame True {
                n150 = call "OUINONV2.vi"("errin"=w421, "image"="Decharge") -> ("error out"=w420:errorcluster, "Booléen"=w422:bool)  [unwired: 8 in]
              }
            }
            n151 = case shown="True" w384 {
              selector: w384 -> [w413 _]
              tunnel: [w413 w416] -> w380
              tunnel: w381 -> [w412 w415]
              tunnel: [w412 w414] -> w379
              frame False {
              }
              frame True {
                n152 = call "OUINONV2.vi"("errin"=w415, "image"="StopLogging") -> ("error out"=w414:errorcluster, "Booléen"=w416:bool)  [unwired: 8 in]
              }
            }
          }
          frame Enabled {
            n153 = call "TENMA_Conf_On.vi"("errin"=w438, "Visa in tenma"=w437) -> ("sortie d'erreur"=w432:errorcluster)  [unwired: 9 in]
            n154 = call "FGV_PDU.vi"("errin"=w432, "Énum"=FGV_Enum."SET", "IN"=TRUE) -> ("errout"=w431:errorcluster)  [unwired: 7 in, 1 out]
            n155 = call <userlib>:"waitXms.vi"("attente (ms)"=u32 600, "errin"=w431) -> ("errout"=w436:errorcluster)  [unwired: 13 in]
            n156 = call "VerifPreDCIR.vi"("errin"=w436, "VISA resource name"=w442) -> ("errout"=w440:errorcluster, "V>35 ?"=w430:bool)  [unwired: 8 in]
            n157 = call <userlib>:"waitXms.vi"("attente (ms)"=u32 600, "errin"=w440) -> ("errout"=w439:errorcluster)  [unwired: 13 in]
            n158 = case shown="True" w430 {
              selector: w430 -> [w449 _]
              tunnel: [w448 w451] -> w446
              tunnel: [w449 w456] -> w445
              tunnel: w444 -> [_ w455]
              tunnel: w443 -> [_ w454]
              tunnel: w439 -> [w448 w458]
              frame False {
                n159 = One Button Dialog(message="Vérifier le branchement de la com, \net que le bouton du tiroir est bien sur DCIR ") -> ()  [unwired: 1 in, 1 out]
              }
              frame True {
                n160 = property on="progression" class="Slide (strict)"(error in=w458, "Visible"=TRUE) -> (error out=w457:errorcluster)  [unwired: 1 in, 1 out]
                n161 = flat-sequence {
                  tunnel: w457 -> [_]
                  frame #0 {
                    n162 = call "FGV_Image.vi"("Énum"=FGV."SET", "IN"="DCIR-EnCours") -> ()  [unwired: 9 in, 1 out]
                  }
                }
                n163 = call "OP500Z8M_ReadFromPDU.vi"("errin"=w457, "SN"=w454, "VISA ITECH Name ?"=w455) -> ("errout"=w450:errorcluster, "BMS OK ?"=w456:bool)  [unwired: 6 in, 1 out]
                n164 = call "FGV_PDU.vi"("errin"=w450, "Énum"=FGV_Enum."SET", "IN"=FALSE) -> ("errout"=w451:errorcluster)  [unwired: 7 in, 1 out]
              }
            }
          }
        }
        n165 = flat-sequence {
          tunnel: [w372] -> w363
          tunnel: w361 -> [w369]
          tunnel: w359 -> [_]
          frame #0 {
            n166 = Select(t=OP500Z8_state."DataDyn" ("Énum"), s=w369, f=OP500Z8_state."GoDCIR" ("cas faux")) -> (s? t:f=w372:T4)
          }
        }
        n167 = property on="progression" class="Slide (strict)"(error in=w351, "Visible"=FALSE, "Value"=0.0 ("progression")) -> (error out=w359:errorcluster)  [unwired: 1 in, 1 out]
      }
      frame "DataDyn" {
        # "Ce VI est en cours...............\nIl faut attendre 3 secondes, si le sub_vi CSV Reader n'a rien comme sortie\n--------------> on passe à l'etape LogErr"
        # "recuperation des donnees du fichier logging"
        n168 = local read "Cluster"() -> (w492:T2)
        n169 = local write "TOP"("Analyse de données" ("TOP")) -> ()
        n170 = Unbundle By Name(w492) -> ("SN"=w489:string)
        n171 = Concatenate Strings("\\\\forseepower.com\\fr\\040 Production\\FR7 - Poitiers\\06 Production\\05. Electronique\\Documents Control lib\\Archives\\ZEN_8\\Contrôle modules\\Controle DCIR", "\\" ("chaîne"), w489, ".csv" ("chaîne")) -> (w476:string)
        n172 = String To Path(string=w476) -> (path=w480:path)
        n173 = global read "VG_DCIR+OUIouNON.vi" "VG_DCIR+ ?"() -> (w462:bool)
        n174 = call "OP500_NEW CSV READER.vi"("errin"=w479, "DCIR+ ?"=w462, "Choisir le fichier CSV"=w480) -> ("sortie d'erreur"=w474:errorcluster, "cluster"=w477:T6)  [unwired: 5 in]
        n175 = local read "Cluster"() -> (w472:T2)
        n176 = call "SubDataDyn.vi"("cluster"=w477, "Cluster en entrée"=w472) -> ("Chaîne"=w482:string, "cluster de sortie"=w471:T7)  [unwired: 8 in]
        n177 = call <userlib>:"Log_basic.vi"("errin"=w488, "date?"=TRUE, "chaîne"=w482, "in"=w486) -> ("sortie d'erreur"=w487:errorcluster, "refnum en sortie"=w485:refnum<file>)  [unwired: 6 in]
        n178 = Unbundle By Name(w471) -> ("VCell Max"=w470:string, "Vcell Min"=w469:string, "NTC Max"=w467:string, "NTC Min"=w468:string)
        n179 = local write "Cluster"(w471) -> ()
        n180 = call "Stall Data Flow.vim"("value in"=w474, "milliseconds to wait"=u32 200) -> ("value out"=w473:errorcluster)  [unwired: 1 out]
        n181 = call "DataDynOK"("NTC Min"=w468, "NTC Max"=w467, "Vcell Min"=w469, "VCell Max"=w470) -> ("DataDynOK ?"=w463:bool)  [unwired: 7 in]
        n182 = Select(t=OP500Z8_state."DTC" ("Next"), s=w463, f=OP500Z8_state."Crash" ("cas faux")) -> (s? t:f=w465:T4)
      }
      frame "DTC" {
        w499 = ";" ("chaîne")
        # "Voir s'il Y a des DTC"
        n183 = local write "TOP"("Analyse les DTC" ("TOP")) -> ()
        n184 = local read "Cluster"() -> (w504:T2)
        n185 = Unbundle By Name(w504) -> ("si DTC"=w498:string)
        n186 = Equal?(x="NO DTC", y=w498) -> (x = y?=w496:bool)
        n187 = call <userlib>:"waitXms.vi"("attente (ms)"=u32 100, "errin"=w502) -> ("errout"=w501:errorcluster)  [unwired: 13 in]
        n188 = Concatenate Strings("DTC" ("chaîne"), w499, w498, w499) -> (w505:string)
        n189 = call <userlib>:"Log_basic.vi"("date?"=TRUE, "chaîne"=w505, "in"=w509) -> ("refnum en sortie"=w508:refnum<file>)  [unwired: 7 in, 1 out]
        n190 = Select(t=OP500Z8_state."DCIR" ("Énum"), s=w496, f=OP500Z8_state."Crash" ("cas faux")) -> (s? t:f=w494:T4)
      }
      frame "DCIR" {
        w519 = ";" ("chaîne")
        # "Recuperation de la valeur DCIR"
        n191 = local write "TOP"("Calcule de la resistance interne" ("TOP")) -> ()
        n192 = local read "Cluster"() -> (w536:T2)
        n193 = global read "VG_DCIR+OUIouNON.vi" "VG_DCIR+ ?"() -> (w516:bool)
        n194 = Unbundle By Name(w536) -> ("DCIR"=w534:string, "DCIR +"=w515:string)
        n195 = call <userlib>:"waitXms.vi"("attente (ms)"=u32 100, "errin"=w528) -> ("errout"=w527:errorcluster)  [unwired: 13 in]
        n196 = Select(t=w515, s=w516, f="NA") -> (s? t:f=w517:string)
        n197 = Concatenate Strings("DCIR-" ("chaîne"), w519, w534, w519, "DCIR+" ("string"), w519, w517, w519) -> (w538:string)
        n198 = Fract/Exp String To Number(string=w534) -> (number=w533:dbl)  [unwired: 3 in, 1 out]
        n199 = call <userlib>:"Log_basic.vi"("errin"=w535, "date?"=TRUE, "chaîne"=w538, "in"=w540) -> ("sortie d'erreur"=w542:errorcluster, "refnum en sortie"=w541:refnum<file>)  [unwired: 6 in]
        n200 = global read "VG_DCIRmax.vi" "DCIRmax"() -> (w524:dbl)
        n201 = global read "VG_DCIRmin.vi" "DCIRmin"() -> (w513:dbl)
        n202 = Increment(x=w513) -> (x+1=w512:dbl)
        n203 = Number To Decimal String(number=w512) -> (decimal integer string=w511:string)  [unwired: 1 in]
        n204 = Select(t=w515, s=w516, f=w511) -> (s? t:f=w514:string)
        n205 = Fract/Exp String To Number(string=w514) -> (number=w525:dbl)  [unwired: 3 in, 1 out]
        n206 = In Range and Coerce(upper limit=w524, x=w533, lower limit=w513) -> (In Range?=w523:bool)  [unwired: 1 out]
        n207 = In Range and Coerce(upper limit=w524, x=w525, lower limit=w513) -> (In Range?=w522:bool)  [unwired: 1 out]
        n208 = And(x=w523, y=w522) -> (x .and. y?=w521:bool)
        n209 = Select(t=OP500Z8_state."Demontage" ("Énum"), s=w521, f=OP500Z8_state."Crash" ("Énum")) -> (s? t:f=w530:T4)
      }
      frame "Demontage" {
        w548 = OP500Z8_state."Next"  # Énum
        n210 = local write "TOP"("Demontage du pack" ("TOP")) -> ()
        n211 = call "OUINONV2.vi"("errin"=w550, "image"="Demontage2" ("IN")) -> ("error out"=w544:errorcluster, "Booléen"=w543:bool)  [unwired: 8 in]
        n212 = Select ("Sélectionner")(t=w548, s=w543, f=OP500Z8_state."Demontage" ("cas faux")) -> (s? t:f=w545:T4)
      }
      frame "Crash" {
        w556 = path "\\\\forseepower.com\\fr/040 Production/FR7 - Poitiers/06 Production/05. Electronique/Documents Control lib/Archives/ZEN_8/Contrôle modules/PV OP500" ("chemin de la cible (utiliser une boîte de dialogue)")
        # "C:\\Users\\ELHAJJ\\OneDrive - FORSEE POWER\\Bureau\\PV ZEN8 TEST"
        n213 = Close File(refnum=w570, error in=w569) -> (path=w559:path, error out=w562:errorcluster)
        n214 = call <userlib>:"waitXms.vi"("attente (ms)"=u32 300, "errin"=w562) -> ("errout"=w560:errorcluster)  [unwired: 13 in]
        n215 = Read from Text File(file (use dialog)=w559, error in=w560) -> (error out=w555:errorcluster)  [unwired: 2 in, 3 out]
        n216 = call "FGV_Image.vi"("Énum"=FGV."SET", "IN"="Crash") -> ()  [unwired: 9 in, 1 out]
        n217 = Copy ("Copier")(8:w555, 10:w556, 11:w559) -> (0:w561:errorcluster)  [unwired: 2 in, 2 out]
        n218 = call "PvgeneratorOP500.vi"("errin"=w561, "network"=w556, "path in"=w559) -> ("sortie d'erreur"=w565:errorcluster, "network out"=w564:path)  [unwired: 5 in, 2 out]
        n219 = call <userlib>:"POP_GOOGLE.vi"("error in"=w565, "chemin"=w564) -> ("error out"=w557:errorcluster)  [unwired: 8 in, 1 out]
        n220 = flat-sequence {
          tunnel: [TRUE] -> w571
          tunnel: w557 -> [_]
          frame #0 {
          }
        }
      }
      frame "Next" {
        w591 = path "\\\\forseepower.com\\fr/040 Production/FR7 - Poitiers/06 Production/05. Electronique/Documents Control lib/Archives/ZEN_8/Contrôle modules/PV OP500" ("chemin de la cible (utiliser une boîte de dialogue)")
        w601 = OP500Z8_state."EXIT"  # Énum
        w602 = OP500Z8_state."Scan"  # Énum
        n221 = global read "VG_DCIR+OUIouNON.vi" "VG_DCIR+ ?"() -> (w576:bool)
        n222 = Select(t="PassNbMP" ("IN"), s=w576, f="PassNbM") -> (s? t:f=w573:string)
        n223 = call "OUINONV2.vi"("errin"=w588, "image"=w573) -> ("error out"=w587:errorcluster, "Booléen"=w586:bool)  [unwired: 8 in]
        n224 = Close File(refnum=w604, error in=w603) -> (path=w594:path, error out=w600:errorcluster)
        n225 = case shown="True" w586 {
          selector: w586 -> [w623 _]
          tunnel: w587 -> [w624 w627]
          tunnel: [w623 w626] -> w584
          tunnel: [w624 w625] -> w583
          frame False {
          }
          frame True {
            n226 = call "OUINONV2.vi"("errin"=w627, "image"="EttJaune" ("IN")) -> ("error out"=w625:errorcluster, "Booléen"=w626:bool)  [unwired: 8 in]
          }
        }
        n227 = call <userlib>:"waitXms.vi"("attente (ms)"=u32 300, "errin"=w600) -> ("errout"=w596:errorcluster)  [unwired: 13 in]
        n228 = Read from Text File(file (use dialog)=w594, error in=w596) -> (error out=w590:errorcluster)  [unwired: 2 in, 3 out]
        n229 = case shown="True" w584 {
          selector: w584 -> [w618 _]
          tunnel: w583 -> [w617 w621]
          tunnel: [w618 w620] -> w585
          tunnel: [w617 w619] -> w582
          frame False {
          }
          frame True {
            n230 = call "OUINONV2.vi"("errin"=w621, "image"="EttBleu" ("IN")) -> ("error out"=w619:errorcluster, "Booléen"=w620:bool)  [unwired: 8 in]
          }
        }
        n231 = case shown="True" w585 {
          selector: w585 -> [w612 _]
          tunnel: w582 -> [w611 w615]
          tunnel: [w612 w614] -> w579
          tunnel: [w611 w613] -> w581
          frame False {
          }
          frame True {
            n232 = call "OUINONV2.vi"("errin"=w615, "image"="eProd" ("IN")) -> ("error out"=w613:errorcluster, "Booléen"=w614:bool)  [unwired: 8 in]
          }
        }
        n233 = Copy ("Copier")(8:w590, 10:w591, 11:w594) -> (0:w595:errorcluster)  [unwired: 2 in, 2 out]
        n234 = call "PvgeneratorOP500.vi"("errin"=w595, "network"=w591, "path in"=w594) -> ("sortie d'erreur"=w598:errorcluster, "network out"=w597:path)  [unwired: 5 in, 2 out]
        n235 = case shown="True" w579 {
          selector: w579 -> [w606 _]
          tunnel: w581 -> [w605 w609]
          tunnel: [w606 w608] -> w578
          tunnel: [w605 w607] -> w580
          frame False {
          }
          frame True {
            n236 = call "OUINONV2.vi"("errin"=w609, "image"="ProdOF" ("IN")) -> ("error out"=w607:errorcluster, "Booléen"=w608:bool)  [unwired: 8 in]
          }
        }
        n237 = call <userlib>:"POP_GOOGLE.vi"("error in"=w598, "chemin"=w597) -> ("error out"=w592:errorcluster)  [unwired: 8 in, 1 out]
        n238 = case shown="True" w578 {
          selector: w578 -> [w630 _]
          tunnel: [w629 w633] -> w577
          tunnel: w580 -> [w629 w631]
          tunnel: [w630 w632] -> w589
          frame False {
          }
          frame True {
            n239 = call "OUINONV2.vi"("errin"=w631, "image"="Next" ("IN")) -> ("error out"=w633:errorcluster, "Booléen"=w632:bool)  [unwired: 8 in]
          }
        }
        n240 = Select(t=w602, s=w589, f=w601) -> (s? t:f=w593:T4)
      }
      frame "EXIT" {
        # "Eteindre le banc avant de quitter labview"
        n241 = call "OUINONV2.vi"("errin"=w640, "image"="TurnOff" ("IN")) -> ("error out"=w639:errorcluster, "Booléen"=w638:bool)  [unwired: 8 in]
        n242 = Select(t=OP500Z8_state."EXIT" ("cas vrai"), s=w638, f=OP500Z8_state."Null" ("Énum")) -> (s? t:f=w636:T4)
        n243 = flat-sequence {
          tunnel: w639 -> [_]
          frame #0 {
            n244 = Quit LabVIEW(quit? (T)=TRUE ("quitter ? (V)")) -> ()
          }
        }
      }
      frame "LogErr" {
        # "En cours.................................................................................................."
        # "au cas ou le fichier de log n'existe pas ou il contient pas le test DCIR"
        n245 = call "OUINONV2.vi"("errin"=w646, "image"="LogErr") -> ("error out"=w647:errorcluster, "Booléen"=w645:bool)  [unwired: 8 in]
        n246 = Select(t=OP500Z8_state."GoDCIR" ("cas vrai"), s=w645, f=OP500Z8_state."Crash" ("Énum")) -> (s? t:f=w648:T4)
      }
    }
    n247 = Wait (ms)(milliseconds to wait=u32 200 ("attente (ms)")) -> ()  [unwired: 1 out]
    n248 = case shown="True" w34 {
      selector: w34 -> [_ w41]
      frame False {
      }
      frame True {
        n249 = local write "STOP"(w41) -> ()
      }
    }
  }
  n250 = while {
    shift-right: [w659] -> _
    shift-left: errorcluster {"status"=FALSE, "code"=0, "source"=""} ("error out") -> [w656]
    stop <- w657 stop-if-true
    # "ici tu met l'image à jour si besoin"
    n251 = Wait (ms)(milliseconds to wait=u32 150 ("attente (ms)")) -> ()  [unwired: 1 out]
    n252 = call "FGV_Image.vi"("Énum"=FGV."GET") -> ("OUT"=w652:string)  [unwired: 10 in]
    n253 = Not Equal?(x=w652, y="") -> (x != y?=w653:bool)
    n254 = case shown="True" w653 {
      tunnel: [w661 w666] -> w659
      tunnel: w656 -> [w661 w665]
      tunnel: w652 -> [_ w664]
      frame False {
      }
      frame True {
        n255 = call <vilib>:"Application Directory.vi"() -> ("Application Directory"=w669:path)
        n256 = Path To String(path=w669) -> (string=w670:string)
        n257 = Concatenate Strings(w670, "\\Image\\" ("chaîne"), w664, ".jpg" ("chaîne")) -> (w668:string)
        n258 = call "FGV_Image.vi"("Énum"=FGV."RAZ") -> ()  [unwired: 10 in, 1 out]
        n259 = String To Path(string=w668) -> (path=w667:path)
        n260 = call <vilib>:"Read JPEG File.vi"("error in (no error)"=w665, "path to JPEG file"=w667) -> ("error out"=w666:errorcluster, "image data"=w673:T8)  [unwired: 7 in, 1 out]
        n261 = call <vilib>:"Draw Flattened Pixmap.vi"("image data"=w673) -> ("new picture"=w662:picture)  [unwired: 8 in]
        n262 = local write "DRAW"(w662) -> ()
      }
    }
    n263 = global read "VG_progressBar.vi" "progression"() -> (→"progression":dbl)
    n264 = global read "VG_Barre_Progression_ISO.vi" "VG_Barre_Progression"() -> (→"Barre de progression ISO":dbl)
    n265 = local read "STOP"() -> (w658:bool)
    n266 = Or(x=w659, y=w658) -> (x .or. y?=w657:bool)
  }
  n267 = while {
    i -> [w676]
    stop <- FALSE stop-if-true
    # "FGV pour led Alarm"
    n268 = Wait (ms)(milliseconds to wait=u32 300) -> ()  [unwired: 1 out]
    n269 = call "OP500Z8_FGV_Alarm.vi"("Énum"=FGV_Enum."GET") -> ("OUT"=w674:bool)  [unwired: 9 in, 1 out]
    n270 = case shown="True" w674 {
      tunnel: w676 -> [_ w679]
      frame False {
      }
      frame True {
        n271 = Quotient & Remainder(x=w679, y=2) -> (x-y*floor(x/y)=w682:i32)  [unwired: 1 out]
        n272 = Not Equal?(x=0, y=w682) -> (x != y?=→"Boolean":bool)
      }
    }
  }
  n273 = disable-structure shown="Enabled" {
    disable-tunnel: [w684 _] -> w4
    frame Enabled {
      n274 = call <userlib>:"PEAK_Init_plus.vi"("Channel"=Channel."PCAN_USBBUS1", "BTR0BTR1"=BaudrateEenum."CAN_BAUD_500K") -> ("errout"=w688:errorcluster, "Channel out"=w687:T9)  [unwired: 8 in]
      n275 = while {
        tunnel: w688 -> [w692]
        tunnel: w687 -> [w697]
        tunnel: [w694] -> w686
        tunnel: [w696] -> w685
        stop <- w695 stop-if-true
        n276 = call "FGV_PDU.vi"("Énum"=FGV_Enum."GET") -> ("OUT"=w698:bool)  [unwired: 9 in, 1 out]
        n277 = case shown="No Error" w692 {
          tunnel: w698 -> [w704 _]
          tunnel: w692 -> [w703 w714]
          tunnel: w697 -> [w702 w713]
          tunnel: [w701 w713] -> w696
          tunnel: [w700 w714] -> w694
          frame No Error {
            n278 = case shown="True" w704 {
              tunnel: w703 -> [w706 w712]
              tunnel: w702 -> [w705 w710]
              tunnel: [w706 w711] -> w700
              tunnel: [w705 w710] -> w701
              frame False {
              }
              frame True {
                n279 = call <userlib>:"PEAK_Can_Write.vi"("CAN Handle"=w710, "MSG type"=enum8{"STD", "RTR", "XTD", "XTD RTR", "STATUS"}."XTD", "errin"=w712, "CAN Data"=u8[] [0, 1, 0, 0, 0, 0, 0, 0], "Identifier"=u32 419401608) -> ("errout"=w711:errorcluster)  [unwired: 6 in]
              }
            }
          }
          frame Error {
          }
        }
        n280 = local read "STOP"() -> (w693:bool)
        n281 = Or(x=w694, y=w693) -> (x .or. y?=w695:bool)
        n282 = Wait (ms) ("Attendre (ms)")(milliseconds to wait=u32 150 ("attente (ms)")) -> ()  [unwired: 1 out]
      }
      n283 = call <userlib>:"CAN Uninitialize.vi"("error in (no error)"=w686, "Channel"=w685) -> ("error out"=w684:errorcluster)  [unwired: 7 in, 2 out]
    }
    frame Disabled {
    }
  }
  n284 = Merge Errors(w26, w25, w4) -> (→"errout":errorcluster)
  n285 = disable-structure shown="Enabled" {
    disable-tunnel: [w715 _] -> _
    frame Disabled {
      n286 = call "Data Dynamiques"() -> ("CMU OK"=w715:bool)  [unwired: 12 in, 7 out]
    }
    frame Enabled {
    }
  }
  "STOP" <- w23
